vi "DefaultPersonality_5774_FPGA_20230215.vi"() -> ()   [LabVIEW 2021, in "GettingStarted_5774_FPGA.lvlib"]
uses:
  GettingStarted_5774_FPGA.lvlib
  <vilib>/Platform/TimedLoop/XDataNode/wakeup.ctl
  <vilib>/Platform/TimedLoop/XDataNode/XDNodeRunTimeDep.lvlib
  <vilib>/Platform/TimedLoop/XDataNode/nitl_modes.ctl
  <vilib>/Platform/TimedLoop/XDataNode/timing_clust.ctl
  <vilib>/Platform/TimedLoop/XDataNode/XDataNode.xnode
  <instrlib>/_niInstr/Streaming/v1/FPGA/niInstr Streaming v1 FPGA.lvlib
  <vilib>/rvi/DataTransferAndStorage/Container/XNode/niFpgaContainer.xnode
  <vilib>/eio/EIONode/EIONode.xnode
  52314b2a-5df6-46e1-8e8c-f4aff1bd7d69.vi
  <instrlib>/FlexRIO/API/FPGA/v1/FlexRIO API FPGA v1.lvlib
  2c54fa2d-4261-47aa-8496-584149bfc8f9.vi
  <vilib>/rvi/interface/RandomDataEmulation/nirviRandomDataFpgaMultiElementTemplate.vi
  <instrlib>/FlexRIO/DRAM FIFO/v2/FPGA/DRAM FIFO/DRAM FIFO v2 FPGA.lvclass
  <instrlib>/_niInstr/Data Formatting/v1/FPGA/niInstr Data Formatting v1 FPGA.lvlib
  <instrlib>/FlexRIO/DRAM FIFO/v2/FPGA/DRAM FIFO/FIFO Depth.ctl
  5b634995-3468-47cf-b53b-988eeb0ffc75.vi
  99fe0684-b2b0-44f8-980b-587ad6a2a500.vi
  <vilib>/rvi/LocalResourceManager/LocalResourceManager.xnode
  <vilib>/rvi/FIFO/Fifo_Resource/niFpgaFifoEmulationRefIn.vi
  <vilib>/rvi/DataTransferAndStorage/Container/Common/niFpgaContainerGetUniqueNameForEmu.vi
  <vilib>/rvi/DataTransferAndStorage/Container/Common/niFpgaContainerSetEmuInfo.vi
  <vilib>/rvi/eio/common/nirviEmuReportErrorAndStop.vi
  <vilib>/rvi/DataTransferAndStorage/Handshake/Emulation/niFpgaHandshakeEmulationRefIn.vi
  <vilib>/rvi/eio/common/nirviEmuTemplateMethod_errors.vi
  <instrlib>/FlexRIO/API/FPGA/v1/Types/Start Trigger IO Resources.ctl
  <instrlib>/FlexRIO/DRAM FIFO/v2/FPGA/DRAM FIFO/Private/DRAM FIFO U256x2/Create 256x2 DRAM FIFO.vi
  <instrlib>/FlexRIO/DRAM FIFO/v2/FPGA/DRAM FIFO/Private/DRAM FIFO U256x2/DRAM FIFO U256x2 v2 FPGA.lvclass
  <instrlib>/FlexRIO/API/FPGA/v1/IO/NI5775/FlexRIO 5775 FPGA v1.lvlib
  <instrlib>/_niInstr/Data Formatting/v1/FPGA/Private/Convert/Boolean Array to U16 Array.vi
  <instrlib>/_niInstr/Data Formatting/v1/FPGA/Private/Convert/U16 array to Boolean Array.vi
  <instrlib>/_niInstr/Streaming/v1/Common/Stream State.ctl
  <instrlib>/_niInstr/Streaming/v1/Common/niInstr Streaming v1 Common.lvlib
panel:
  out "flexrio.trigger.start.metadata 0":u16
  in  "flexrio.io.interleaving factor 0":u16=1
  out "flexrio.module.dram ready 0":bool
  in  "flexrio.buffer.fifo.reset 0":bool
  out "flexrio.module.io ready 0":bool
  out "flexrio.module.io error 0":i32
  out "flexrio.module.data valid 0":bool
  in  "flexrio.stream.channels enabled 0":u64 caption="stream.num samples 0"
  in  "flexrio.buffer.delay.clocks 0":u16=1
  in  "flexrio.buffer.delay.reset 0":bool
  in  "flexrio.trigger.analog.edge.rising 0":bool=TRUE
  in  "flexrio.trigger.analog.edge.hysteresis 0":fxp<+/-,32,1>
  in  "flexrio.trigger.analog.edge.threshold 0":fxp<+/-,32,1>
  in  "User-defined Start Trigger - AI":bool
  in  "flexrio.trigger.start.cfg 0":u16
  in  "flexrio.trigger.analog.edge.channel 0":fxp<+,2,2> format="%#_4g"
  in  "stream.num samples 0":u64
  in  "stream.request state 0":T1
  out "stream.state 0":T1
  out "stream.samples transferred 0":u64
  out "stream.metadata 0":u64
  # "Device Utilization\n---------------------------\nTotal Slices: 53.9% (16318 out of 30300)\nSlice Registers: 20.4% (98957 out of 484800)\nSlice LUTs: 33.5% (81283 out of 242400)\nBlock RAMs: 40.5% (243 out of 600)\nDSP48s: 0.4% (8 out of 1920)\n\nNote: Utilization numbers are for the KU040. Exact values will vary for the KU060 and KU035."
  # "Data Path Configuration"
  # "AI Trigger Configuration"
  # "AI Stream Configuration"
  # "Module Status"
  # "User-defined Controls"
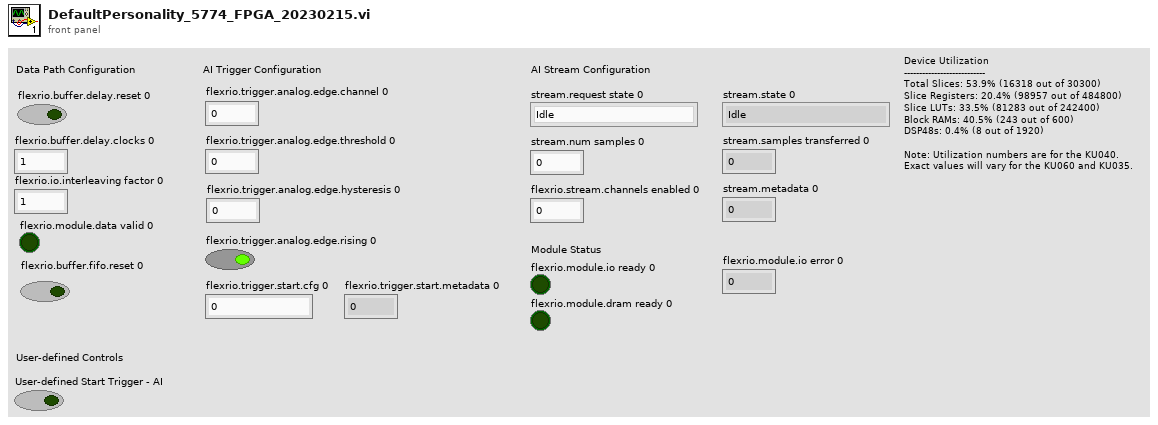
[diagram p1: front panel]
types:
  T1 = typedef "niInstr Streaming v1 Common.lvlib/Stream State.ctl" = enum8{"Idle", "Finite Transfer", "Continuous", "Done", "Error", "Not Ready", "Cancel"}
  T2 = typedef "DRAM FIFO v2 FPGA.lvclass/FIFO Depth.ctl" = u8
  T3 = typedef "XDNodeRunTimeDep.lvlib/timing_clust.ctl" = cluster{"Expected End [f-1]":u64, "Actual End [f-1]":u64, "Finished Late? [f-1]":bool, "Expected End [i-1]":u64, "Actual End [i-1]":u64, "Finished Late? [i-1]":bool, "Expected Start [i]":u64, "Actual Start [i]":u64, "Expected Start [f]":u64, "Actual Start [f]":u64, "Source Name":string, "Structure Name":string, "Period":i64, "Deadline":i64, "Offset":i64, "Start":i64, "Priority":i32, "Timeout":i32, "Mode":T4, "Wakeup Reason":T5, "Error":errorcluster, "Source Type":string, "Secondary Source Type":string, "Global End Time":u64, "Global Start Time":u64, "Frame Duration":u64, "Iteration Duration":u64, "Assigned CPU":i32, "I/O Scan Engine Mode":u32}
  T4 = typedef "XDNodeRunTimeDep.lvlib/nitl_modes.ctl" = enum32{"No Change", "Process missed periods, maintain original phase", "Discard missed periods, maintain original phase", "Process missed periods, ignore original phase", "Discard missed periods, ignore original phase"}
  T5 = typedef "XDNodeRunTimeDep.lvlib/wakeup.ctl" = enum32{"Normal", "Aborted", "Asynchronous wakeup", "Timing source error", "Timed loop error", "Timeout"}
  T6 = typedef "FlexRIO API FPGA v1.lvlib/Start Trigger IO Resources.ctl" = cluster{"start trigger":refnum<k21>, "started event":refnum<k21>, "start trigger for export":refnum<k21>, "start trigger for tclk":refnum<k21>}
  T7 = typedef "FlexRIO API FPGA v1.lvlib/Start Trigger Control.ctl" = cluster{"arm start":bool, "done":bool}
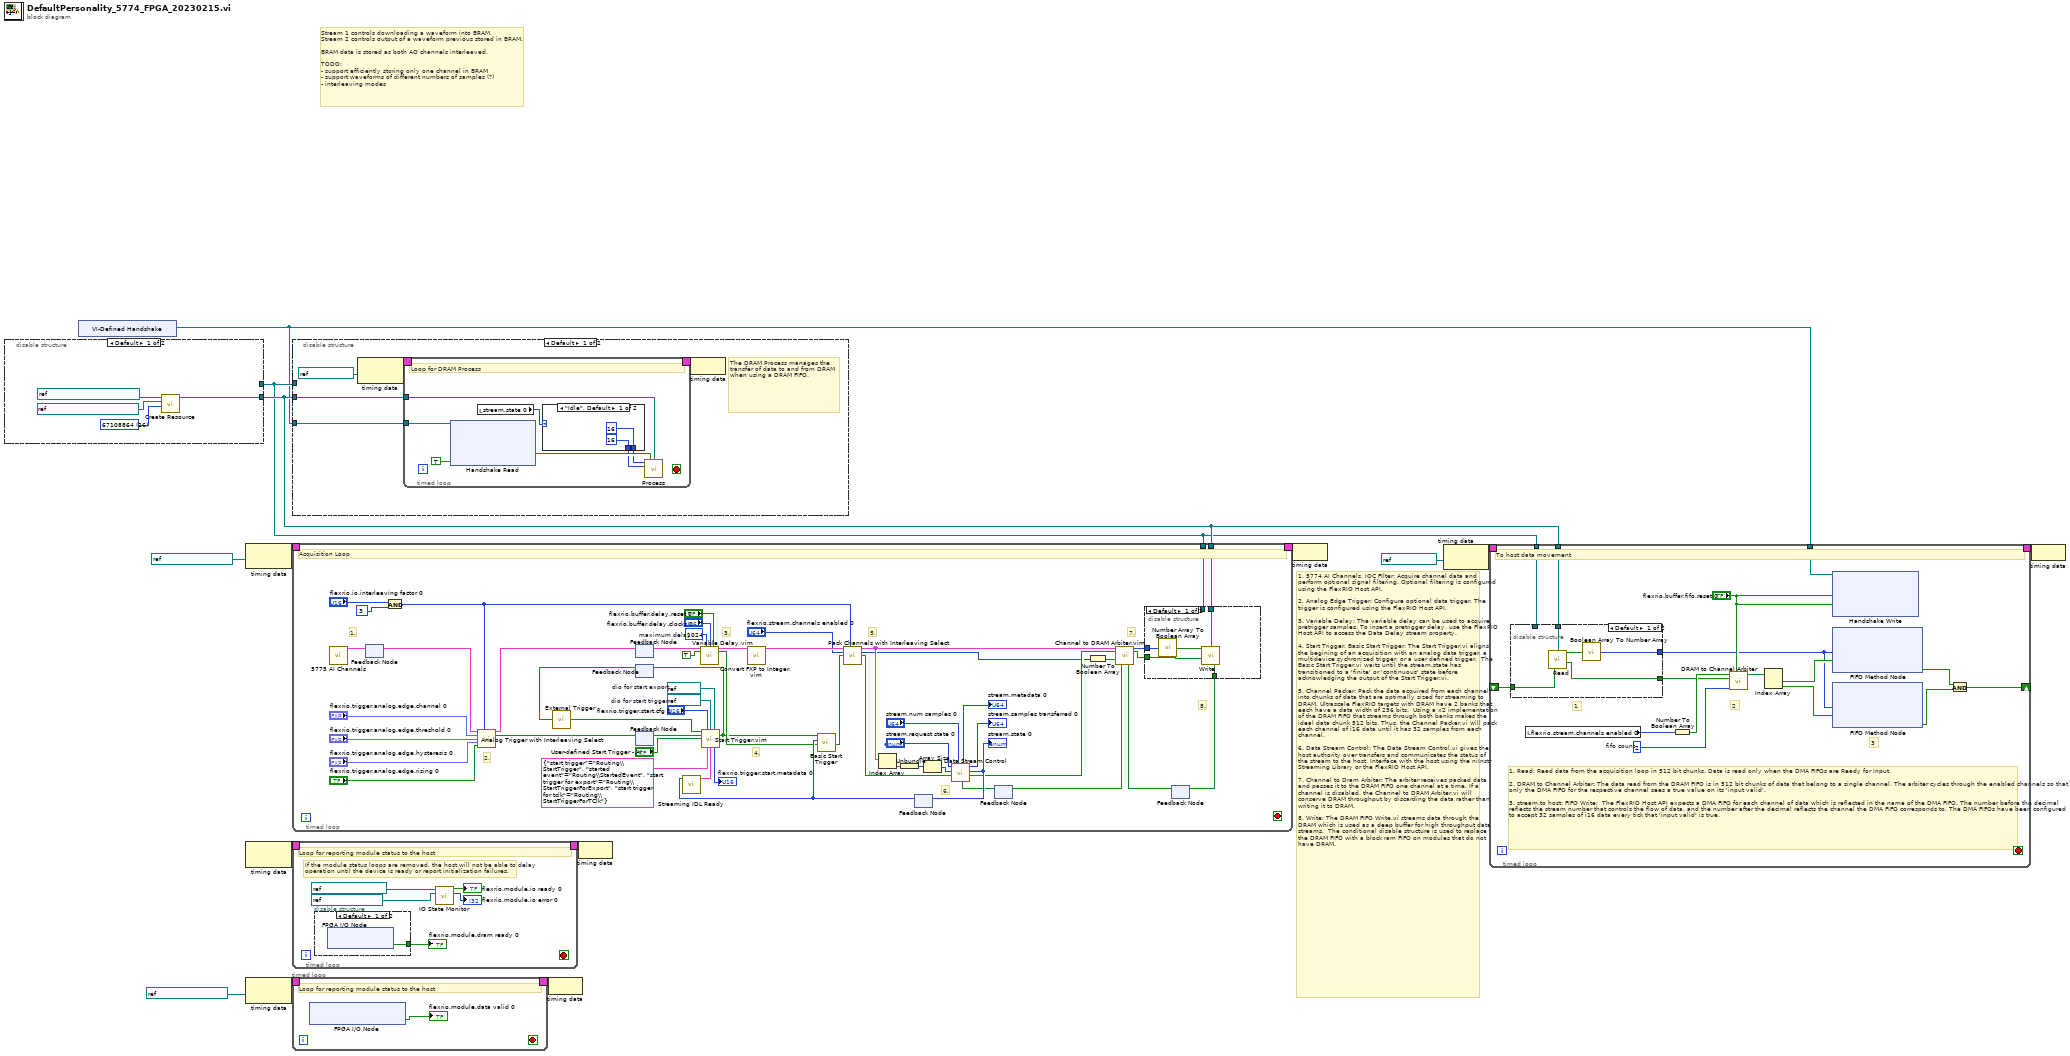
[diagram p0: block diagram]
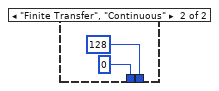
[diagram p2: hidden frame]
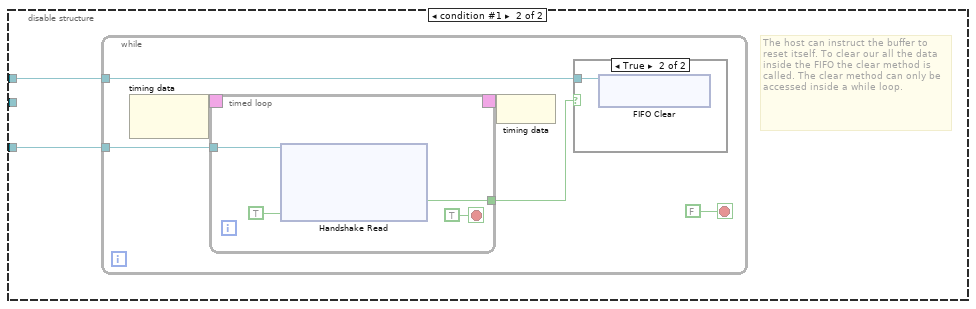
[diagram p3: hidden frame]
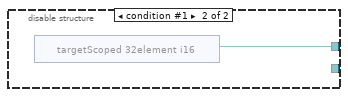
[diagram p5: hidden frame]
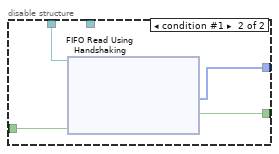
[diagram p6: hidden frame]
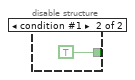
[diagram p7: hidden frame]
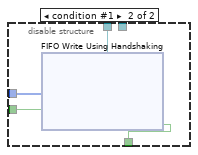
[diagram p8: hidden frame]
diagram:
  # "Stream 1 controls downloading a waveform into BRAM.\nStream 2 controls output of a waveform previous stored in BRAM.\n\nBRAM data is stored as both AO channels interleaved.\n\nTODO:\n- support efficiently storing only one channel in BRAM\n- support waveforms of different numbers of samples (?)\n- interleaving modes"
  # "1. 5774 AI Channels, IOC FIlter: Acquire channel data and perform optional signal filtering. Optional filtering is configured using the FlexRIO Host API.\n\n2. Analog Edge Trigger: Configure optional data trigger. The trigger is configured using the FlexRIO Host API.\n\n3. Variable Delay: The variable delay can be used to acquire pretrigger samples. To insert a pretrigger delay, use the FlexRIO Host API to access the Data Delay stream property. \n\n4. Start Trigger, Basic Start Trigger: The Start Trigger.vi aligns the begining of an acquisition with an analog data trigger, a multidevice sychronized trigger, or a user defined trigger.  The Basic Start Trigger.vi waits until the stream.state has transitioned to a 'finite' or 'continuous' state before acknowledging the output of the Start Trigger.vi.\n\n5. Channel Packer: Pack the data acquired from each channel into chunks of data that are optimally sized for streaming to DRAM. Ultrascale FlexRIO targets with DRAM have 2 banks that each have a data width of 256 bits.  Using a x2 implementation of the DRAM FIFO that streams through both banks makes the ideal data chunk 512 bits. Thus, the Channel Packer.vi will pack each channel of i16 data until it has 32 samples from each channel. \n\n6. Data Stream Control: The Data Stream Control.vi gives the host authority over transfers and communicates the status of the stream to the host. Interface with the host using the niInstr Streaming Library or the FlexRIO Host API. \n\n7. Channel to Dram Arbiter: The arbiter receives packed data and passes it to the DRAM FIFO one channel at a time. If a channel is disabled, the Channel to DRAM Arbiter.vi will conserve DRAM throughput by discarding the data rather than writing it to DRAM. \n\n8. Write: The DRAM FIFO Write.vi streams data through the DRAM which is used as a deep buffer for high throughput data streams.  The conditional disable structure is used to replace the DRAM FIFO with a block ram FIFO on modules that do not have DRAM."
  n1 = disable-structure shown="Default" {
    disable-tunnel: [w18 _] -> w6
    disable-tunnel: [_ w19] -> w5
    frame condition #0 (active) {
      w15 = T2 26 items=["4"=2, "8"=3, "16"=4, "32"=5, "64"=6, "128"=7, "256"=8, "512"=9, "1024"=10, "2048"=11, "4096"=12, "8192"=13, "16384"=14, "32768"=15, "65536"=16, "131072"=17, "262144"=18, "524288"=19, "1048576"=20, "2097152"=21, "4194304"=22, "8388608"=23, "16777216"=24, "33554432"=25, "67108864"=26, "134217728"=27, "268435456"=28, "536870912"=29, "1073741824"=30, "2147483648"=31, "4294967296"=32] ("actual # of DRAM elements")
      n2 = call-poly <instrlib>:"Create Resource.vi"("actual # of DRAM elements"=w15, "memory refnum 2"=refnum<k21> "DRAM FIFO Bank1 67108864" ("memory refnum"), "memory refnum"=refnum<k21> "DRAM FIFO Bank0 67108864") -> ("DRAM FIFO ref out"=w18:refnum<class "DRAM FIFO v2 FPGA.lvclass">)  [unwired: 8 in]
    }
    frame condition #1 {
      n3 = xnode "targetScoped 32element i16"() -> ("FIFO Out"=w19:refnum<k21>)
    }
  }
  n4 = xnode "VI-Defined Handshake"() -> ("Handshake Out"=w4:refnum<k21>)
  n5 = node-c288(refnum<k21> "IO Socket\\Data Clock" ("Source Name")) -> (w14:T3)
  n6 = node-c288() -> (w11:T3)  [unwired: 1 in]
  n7 = node-c288(refnum<k21> "IO Socket\\Data Clock" ("Source Name")) -> (w3:T3)
  n8 = disable-structure shown="Default" {
    disable-tunnel: w6 -> [w21 _]
    disable-tunnel: w5 -> [_ w43]
    disable-tunnel: w4 -> [w20 w42]
    frame condition #0 (active) {
      # "The DRAM Process manages the transfer of data to and from DRAM when using a DRAM FIFO."
      n9 = node-c288(refnum<k21> "DRAM Clock" ("Source Name")) -> (w24:T3)
      n10 = timed-loop {
        timing: w24 -> [_]
        timing-out: [_] -> w23
        tunnel: w21 -> [w31]
        tunnel: w20 -> [w30]
        stop <- _ stop-if-true
        # "Loop for DRAM Process"
        n11 = xnode ("Handshake Read")("Ready for Output"=TRUE, "Handshake In"=w30) -> ("Output Valid"=w28:bool)  [unwired: 2 out]
        n12 = local read "stream.state 0"() -> (w27:T1)
        n13 = case shown="\"Idle\", Default" w27 {
          tunnel: [u16 16 ("write grant time (clock ticks)") u16 128 ("write grant time (clock ticks)")] -> w26
          tunnel: [u16 16 ("read grant time (clock ticks)") u16 0 ("read grant time (clock ticks)")] -> w25
          frame "Idle", Default {
          }
          frame "Finite Transfer", "Continuous" {
          }
        }
        n14 = call <instrlib>:"Process.vi"("write grant time (clock ticks)"=w26, "reset DRAM"=w28, "DRAM FIFO ref in"=w31, "read grant time (clock ticks)"=w25) -> ()  [unwired: 10 in, 2 out]
      }
      n15 = node-c288(w23) -> ()
    }
    frame condition #1 {
      # "The host can instruct the buffer to reset itself. To clear our all the data inside the FIFO the clear method is called. The clear method can only be accessed inside a while loop."
      n16 = while {
        tunnel: w43 -> [w49]
        tunnel: w42 -> [w48]
        stop <- FALSE stop-if-true
        n17 = node-c288() -> (w45:T3)  [unwired: 1 in]
        n18 = timed-loop {
          timing: w45 -> [_]
          timing-out: [_] -> w44
          tunnel: w48 -> [w53]
          tunnel: [w51] -> w46
          stop <- TRUE stop-if-true
          n19 = xnode ("Handshake Read")("Ready for Output"=TRUE, "Handshake In"=w53) -> ("Output Valid"=w51:bool)  [unwired: 2 out]
        }
        n20 = node-c288(w44) -> ()
        n21 = case shown="True" w46 {
          tunnel: w49 -> [_ w58]
          frame False {
          }
          frame True {
            n22 = xnode ("FIFO Clear")("FIFO In"=w58) -> ()  [unwired: 1 out]
          }
        }
      }
    }
  }
  n23 = timed-loop {
    timing: w14 -> [_]
    timing-out: [_] -> w13
    tunnel: w6 -> [w86]
    tunnel: w5 -> [w85]
    stop <- _ stop-if-true
    w99 = u16 1024  # maximum delay
    w104 = refnum<k21> "DIO 0"  # dio for start trigger
    w103 = refnum<k21> "DIO 1"  # dio for start export
    # "5."
    # "2."
    # "8."
    # "7."
    # "6."
    # "4."
    # "3."
    # "1."
    # "Acquisition Loop"
    n24 = call <instrlib>:"5775 AI Channels.vi"() -> ("all channels"=w63:cluster{fxp<+/-,12,1>[]}[])  [unwired: 15 in]
    n25 = feedback #1() -> (w62:cluster{fxp<+/-,12,1>[]}[])  [unwired: 1 in]
    n26 = feedback-in #1(w63) -> ()
    n27 = And(x="flexrio.io.interleaving factor 0", y=u16 3) -> (x .and. y?=w68:u16)
    n28 = call "Analog Trigger with Interleaving Select.vi"("all channels"=w62, "interleaving factor"=w68, "channel"="flexrio.trigger.analog.edge.channel 0", "trigger level"="flexrio.trigger.analog.edge.threshold 0", "hysteresis level"="flexrio.trigger.analog.edge.hysteresis 0", "rising edge"="flexrio.trigger.analog.edge.rising 0") -> ("all channels delayed"=w59:cluster{fxp<+/-,12,1>[]}[], "triggered"=w81:bool)  [unwired: 8 in]
    n29 = feedback #2() -> (w98:cluster{fxp<+/-,12,1>[]}[])  [unwired: 1 in]
    n30 = feedback-in #2(w59) -> ()
    n31 = feedback #3() -> (w60:bool)  [unwired: 1 in]
    n32 = call "External Trigger.vi"("front panel trigger out"=w60) -> ("front panel trigger in"=w65:bool)  [unwired: 4 in]
    n33 = feedback-in #4(w81) -> ()
    n34 = feedback #4() -> (w101:bool)  [unwired: 1 in]
    n35 = call "Variable Delay.vim"("Array in"=w98, "maximum delay"=w99, "delay"="flexrio.buffer.delay.clocks 0", "reset"="flexrio.buffer.delay.reset 0", "data valid"=TRUE) -> ("Array out"=w92:cluster{fxp<+/-,12,1>[]}[], "data valid?"=w97:bool)  [unwired: 8 in, 1 out]
    n36 = call "Convert FXP to Integer.vim"("Array in"=w92) -> ("Array"=w76:cluster{i16[]}[])  [unwired: 14 in]
    n37 = feedback #5() -> (w102:T1)  [unwired: 1 in]
    n38 = call <instrlib>:"Streaming IDL Ready.vi"("stream.state"=w102) -> ("start trigger control"=w106:T7)  [unwired: 10 in]
    n39 = call "Start Trigger.vim"("external analog trigger"=w65, "flexrio.trigger.start.cfg 0"="flexrio.trigger.start.cfg 0", "dio start"=w104, "dio for start export"=w103, "analog trigger"=w101, "user-defined start trigger"="User-defined Start Trigger - AI", "trigger io resources"=T6 {"start trigger"="Routing\\StartTrigger", "started event"="Routing\\StartedEvent", "start trigger for export"="Routing\\StartTriggerForExport", "start trigger for tclk"="Routing\\StartTriggerForTClk"}, "start trigger control"=w106) -> ("conditioned start trigger"=w61:bool, "flexrio.trigger.start.metadata 0"=→"flexrio.trigger.start.metadata 0":u16)  [unwired: 5 in, 1 out]
    n40 = feedback-in #3(w61) -> ()
    n41 = call <instrlib>:"Basic Start Trigger.vi"("data valid?"=w97, "stream.state"=w102, "start trigger"=w61) -> ("data valid"=w74:bool)  [unwired: 8 in]
    n42 = call "Pack Channels with Interleaving Select.vi"("Array"=w76, "interleaving factor"=w68, "channels enabled"="flexrio.stream.channels enabled 0", "data valid?"=w74) -> ("Array out"=w75:cluster{i16[]}[], "channels enabled out"=w72:u64, "data valid"=w73:bool)  [unwired: 9 in]
    n43 = Index Array(array=w75) -> (element=w94:cluster{i16[]})  [unwired: 1 in]
    n44 = Unbundle(w94) -> (w93:i16[])
    n45 = Array Size(array=w93) -> (size(s)=w112:i32)
    n46 = feedback #6() -> (w82:bool)  [unwired: 1 in]
    n47 = call <instrlib>:"Data Stream Control.vi"("ready for input?"=w82, "stream.num samples 0"="stream.num samples 0", "data valid"=w73, "element count"=w112, "stream.request state 0"="stream.request state 0") -> ("send data"=w89:bool, "stream.state 0"=w107:T1, "stream.samples transferred 0"=→"stream.samples transferred 0":u64, "stream.metadata 0"=→"stream.metadata 0":u64)  [unwired: 2 in, 1 out]
    "stream.state 0" <- w107
    n48 = feedback-in #5(w107) -> ()
    n49 = Number To Boolean Array(number=w72) -> (Boolean array=w90:bool[])
    n50 = feedback #7() -> (w84:bool)  [unwired: 1 in]
    n51 = call "Channel to DRAM Arbiter.vim"("channels in"=w75, "valid in"=w89, "channels enabled"=w90, "ready for output"=w84) -> ("data"=w91:i16[], "valid out"=w87:bool, "ready for input"=w83:bool)  [unwired: 9 in]
    n52 = feedback-in #6(w83) -> ()
    n53 = disable-structure shown="Default" {
      disable-tunnel: w91 -> [w117 w120]
      disable-tunnel: [w115 w118] -> w88
      disable-tunnel: w87 -> [w114 w119]
      disable-tunnel: w86 -> [w113 _]
      disable-tunnel: w85 -> [_ w121]
      frame condition #0 (active) {
        n54 = call-poly <instrlib>:"Number Array To Boolean Array.vi"("data in"=w117) -> ("data out"=w116:bool[])  [unwired: 14 in]
        n55 = call <instrlib>:"Write.vi"("element"=w116, "DRAM FIFO ref in"=w113, "input valid"=w114) -> ("ready for input"=w115:bool)  [unwired: 12 in]
      }
      frame condition #1 {
        n56 = xnode ("FIFO Write Using Handshaking")("Element"=w120, "Input Valid"=w119, "FIFO In"=w121) -> ("Ready for Input"=w118:bool)  [unwired: 1 out]
      }
    }
    n57 = feedback-in #7(w88) -> ()
  }
  n58 = timed-loop {
    timing: w11 -> [_]
    timing-out: [_] -> w10
    stop <- _ stop-if-true
    # "If the module status loops are removed, the host will not be able to delay operation until the device is ready or report initialization failures."
    # "Loop for reporting module status to the host"
    n59 = disable-structure shown="Default" {
      disable-tunnel: [w129 TRUE ("flexrio.module.dram ready 0")] -> w126
      frame condition #0 (active) {
        n60 = xnode "FPGA I/O Node"() -> ("DRAM Ready"=w129:bool)  [unwired: 1 in, 1 out]
      }
      frame condition #1 {
      }
    }
    "flexrio.module.dram ready 0" <- w126
    n61 = call <instrlib>:"IO State Monitor.vi"("io error resource"=refnum<k21> "IO Socket\\IO Error" ("FPGA I/O In"), "io ready resource"=refnum<k21> "IO Socket\\IO Ready" ("FPGA I/O In")) -> ("flexrio.module.io error 0"=→"flexrio.module.io error 0":i32, "flexrio.module.io ready 0"=→"flexrio.module.io ready 0":bool)  [unwired: 8 in]
  }
  n62 = timed-loop {
    timing: w3 -> [_]
    timing-out: [_] -> w2
    stop <- _ stop-if-true
    # "Loop for reporting module status to the host"
    n63 = xnode "FPGA I/O Node"() -> ("IO Socket\\AI Data Valid"=→"flexrio.module.data valid 0":bool)  [unwired: 1 in, 1 out]
  }
  n64 = node-c288(w2) -> ()
  n65 = node-c288(w10) -> ()
  n66 = node-c288(w13) -> ()
  n67 = node-c288(refnum<k21> "PXIe_CLK200" ("Source Name")) -> (w9:T3)
  n68 = timed-loop {
    timing: w9 -> [_]
    timing-out: [_] -> w8
    tunnel: w6 -> [w150]
    shift-right: [w141] -> _
    shift-left: _ -> [w149]
    tunnel: w5 -> [w148]
    tunnel: w4 -> [w147]
    stop <- _ stop-if-true
    w143 = 2  # fifo count
    # "3"
    # "2"
    # "1. Read: Read data from the acquisition loop in 512 bit chunks. Data is read only when the DMA FIFOs are Ready for Input.\n\n2. DRAM to Channel Arbiter: The data read from the DRAM FIFO is in 512 bit chunks of data that belong to a single channel. The arbiter cycles through the enabled channels so that only the DMA FIFO for the respective channel sees a true value on its 'input valid'. \n\n3. stream.to host: FIFO Write:  The FlexRIO Host API expects a DMA FIFO for each channel of data which is reflected in the name of the DMA FIFO. The number before the decimal reflects the stream number that controls the flow of data, and the number after the decimal reflects the channel the DMA FIFO corresponds to. The DMA FIFOs have been configured to accept 32 samples of i16 data every tick that 'input valid' is true."
    # "1"
    # "To host data movement"
    n69 = disable-structure shown="Default" {
      disable-tunnel: w150 -> [w156 _]
      disable-tunnel: [w155 w158] -> w144
      disable-tunnel: [w154 w159] -> w138
      disable-tunnel: w149 -> [w152 w157]
      disable-tunnel: w148 -> [_ w160]
      frame condition #0 (active) {
        n70 = call <instrlib>:"Read.vi"("DRAM FIFO ref in"=w156, "ready for output"=w152) -> ("element"=w153:bool[], "output valid"=w155:bool)  [unwired: 12 in]
        n71 = call-poly <instrlib>:"Boolean Array To Number Array.vi"("data in"=w153) -> ("data out"=w154:u16[])  [unwired: 14 in]
      }
      frame condition #1 {
        n72 = xnode ("FIFO Read Using Handshaking")("Ready for Output"=w157, "FIFO In"=w160) -> ("Element"=w159:i16[], "Output Valid"=w158:bool)  [unwired: 1 out]
      }
    }
    n73 = local read "flexrio.stream.channels enabled 0"() -> (w151:u64)
    n74 = Number To Boolean Array(number=w151) -> (Boolean array=w145:bool[])
    n75 = call <instrlib>:"DRAM to Channel Arbiter.vi"("reset"="flexrio.buffer.fifo.reset 0", "channel count"=w143, "input valid"=w144, "channels enabled"=w145) -> ("valid channel"=w146:bool[])  [unwired: 6 in, 1 out]
    n76 = Index Array(array=w146) -> (element #1=w140:bool, element #2=w139:bool)  [unwired: 2 in]
    n77 = xnode ("Handshake Write")("Data"="flexrio.buffer.fifo.reset 0", "Input Valid"="flexrio.buffer.fifo.reset 0", "Handshake In"=w147) -> ()  [unwired: 2 out]
    n78 = xnode ("FIFO Method Node")("Element"=w138, "Input Valid"=w140) -> ("Ready for Input"=w136:bool)  [unwired: 1 in, 1 out]
    n79 = xnode ("FIFO Method Node")("Element"=w138, "Input Valid"=w139) -> ("Ready for Input"=w137:bool)  [unwired: 1 in, 1 out]
    n80 = And(x=w136, y=w137) -> (x .and. y?=w141:bool)
  }
  n81 = node-c288(w8) -> ()
